vi "Review.vi"() -> ()   [LabVIEW 2023]
uses:
  <vilib>/measure/madcrms.llb/Basic Averaged DC-RMS for N Chan.vi
  <vilib>/measure/NI_MAPro.lvlib
panel:
  out "Mains Request":sgl
  out "Bus Current Load Demand":dbl
  out "Bus Voltage RMS/100":dbl
  out "Bus Current Demand to SM":dynamicdata(graph)
  out "Battery Charge Sw":bool
  out "Battery Discharge Sw":bool
  out "LoadSw3":bool
  out "LoadSw2":bool
  out "LoadSw1":bool
  out "SM PV Current":dbl
  out "SM Wind Current":dbl
  out "Bus Current (rms)":dynamicdata(graph)
  out "Bus Voltage (rms)":dynamicdata(graph)
  out "Load 3":bool
  out "Load 2":bool
  out "Load 1":bool
  out "Charge Batt":bool
  out "Discharge Batt":bool
  out "Analog Input (Main Capacity 0-10V)":dynamicdata(graph)
  in  "stop":bool
  out "Voltage Dip Supply < Demand":dynamicdata(graph)
  out "240 Vrms Supply >=Demand":dynamicdata(graph)
  out "Capacity - Demand (current)":dynamicdata(graph)
  in  "Battery Charging Current":dbl
  in  "Battery Disharging Current":dbl
  in  "Load 3 Demand (current)":dbl
  in  "Load 2 Demand (current)":dbl
  in  "Load 1 Demand (current)":dbl
  out "Battery Charging Current":dynamicdata(graph)
  out "Load 3 Current":dynamicdata(graph)
  out "Load 2 Current":dynamicdata(graph)
  out "Load 1 Current":dynamicdata(graph)
  out "Battery Discharging Current (A rms)":dynamicdata(graph)
  out "Main Available Current (A rms)":dynamicdata(graph)
  out "PV Available Current (A rms)":dynamicdata(graph)
  out "Wind Available Current (A rms)":dynamicdata(graph)
  in  "Main capacity (current)":dbl
  in  "Max PV capacity (current)":dbl
  in  "Max wind capacity (current)":dbl
  out "Bus Voltage 240Vrms/100":dynamicdata(graph)
  # "Smart Meter Emulator Algorithm inputs and output status"
  # "Final Review Software using software algorithm and profile inputs - produces output file for submission  - by Russel Torah - 2021"
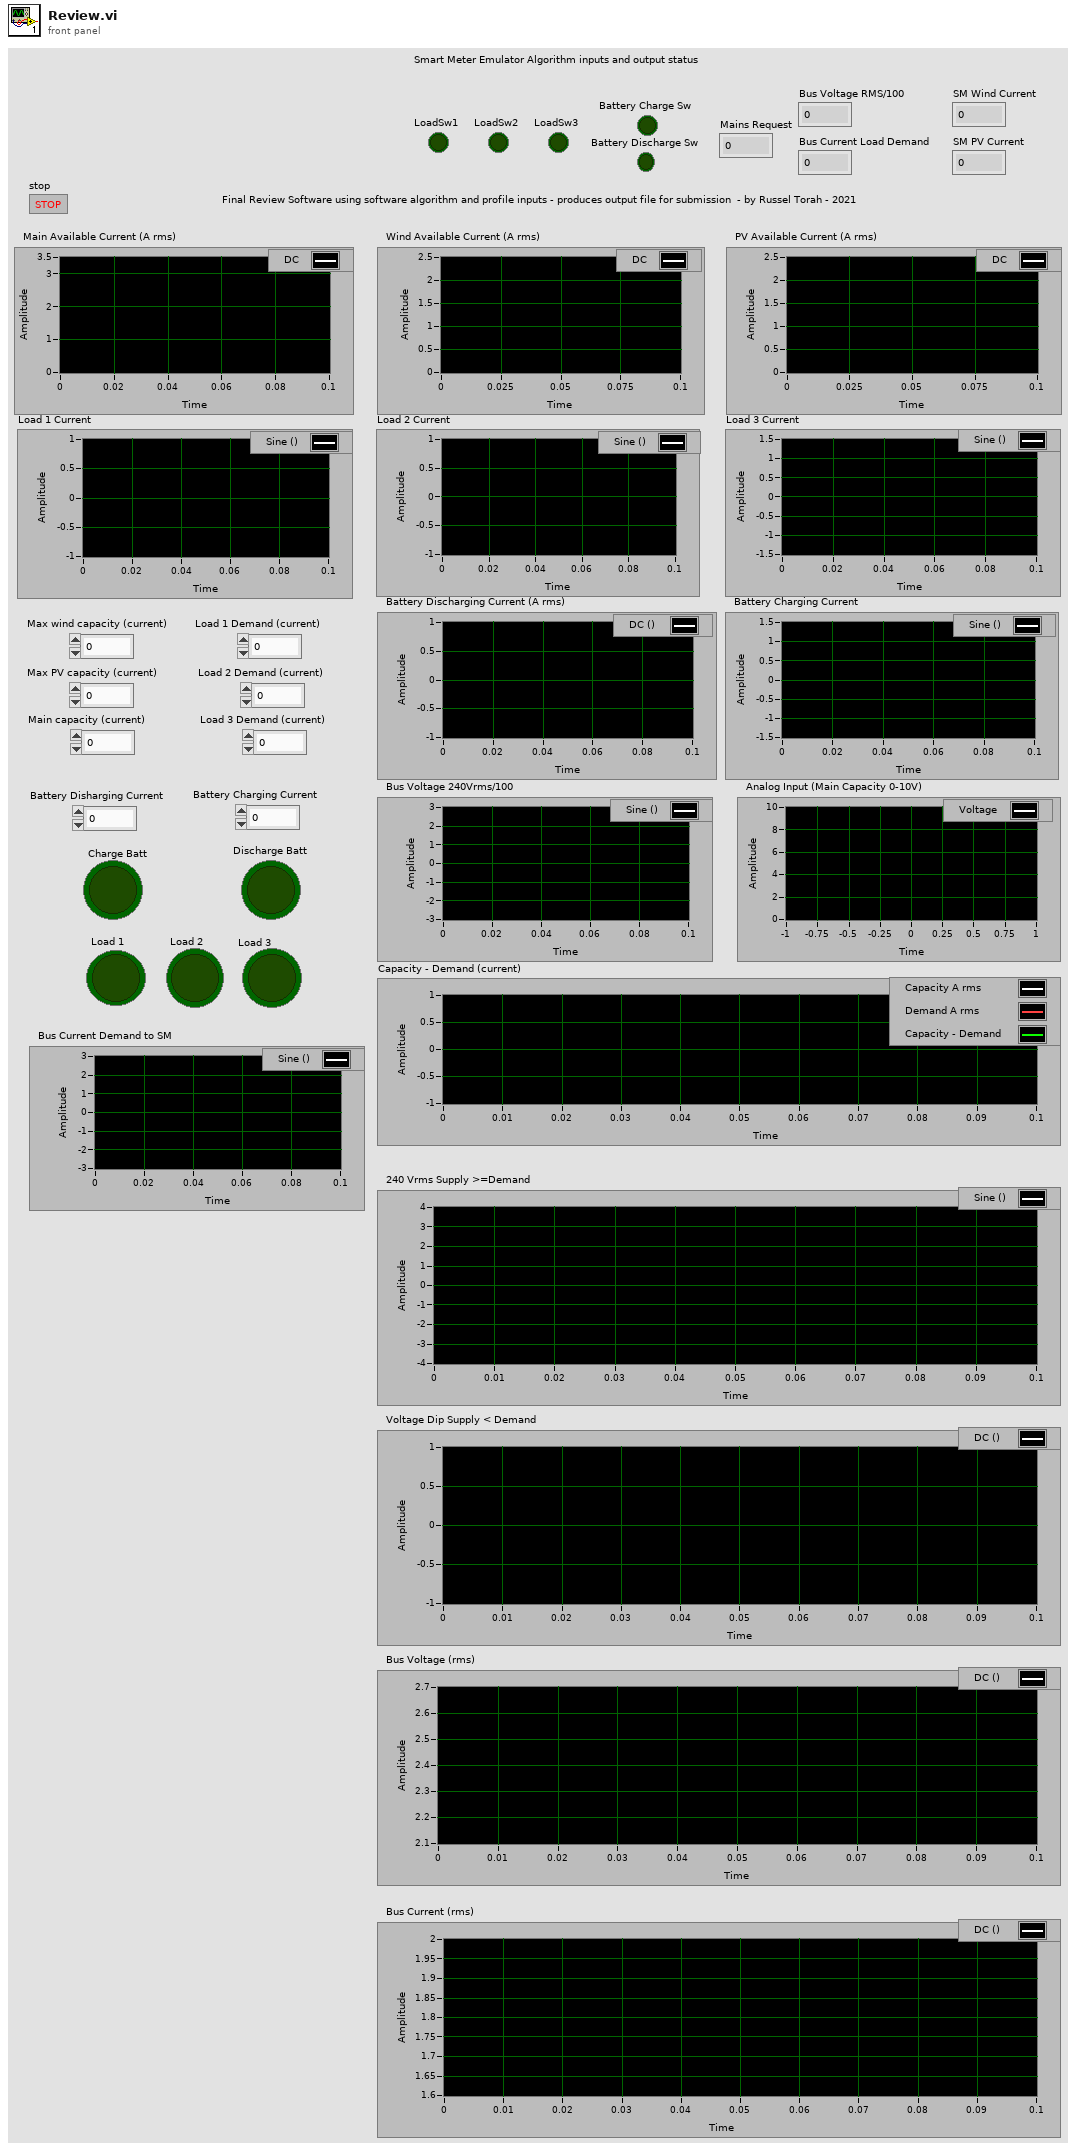
[diagram p1: front panel]
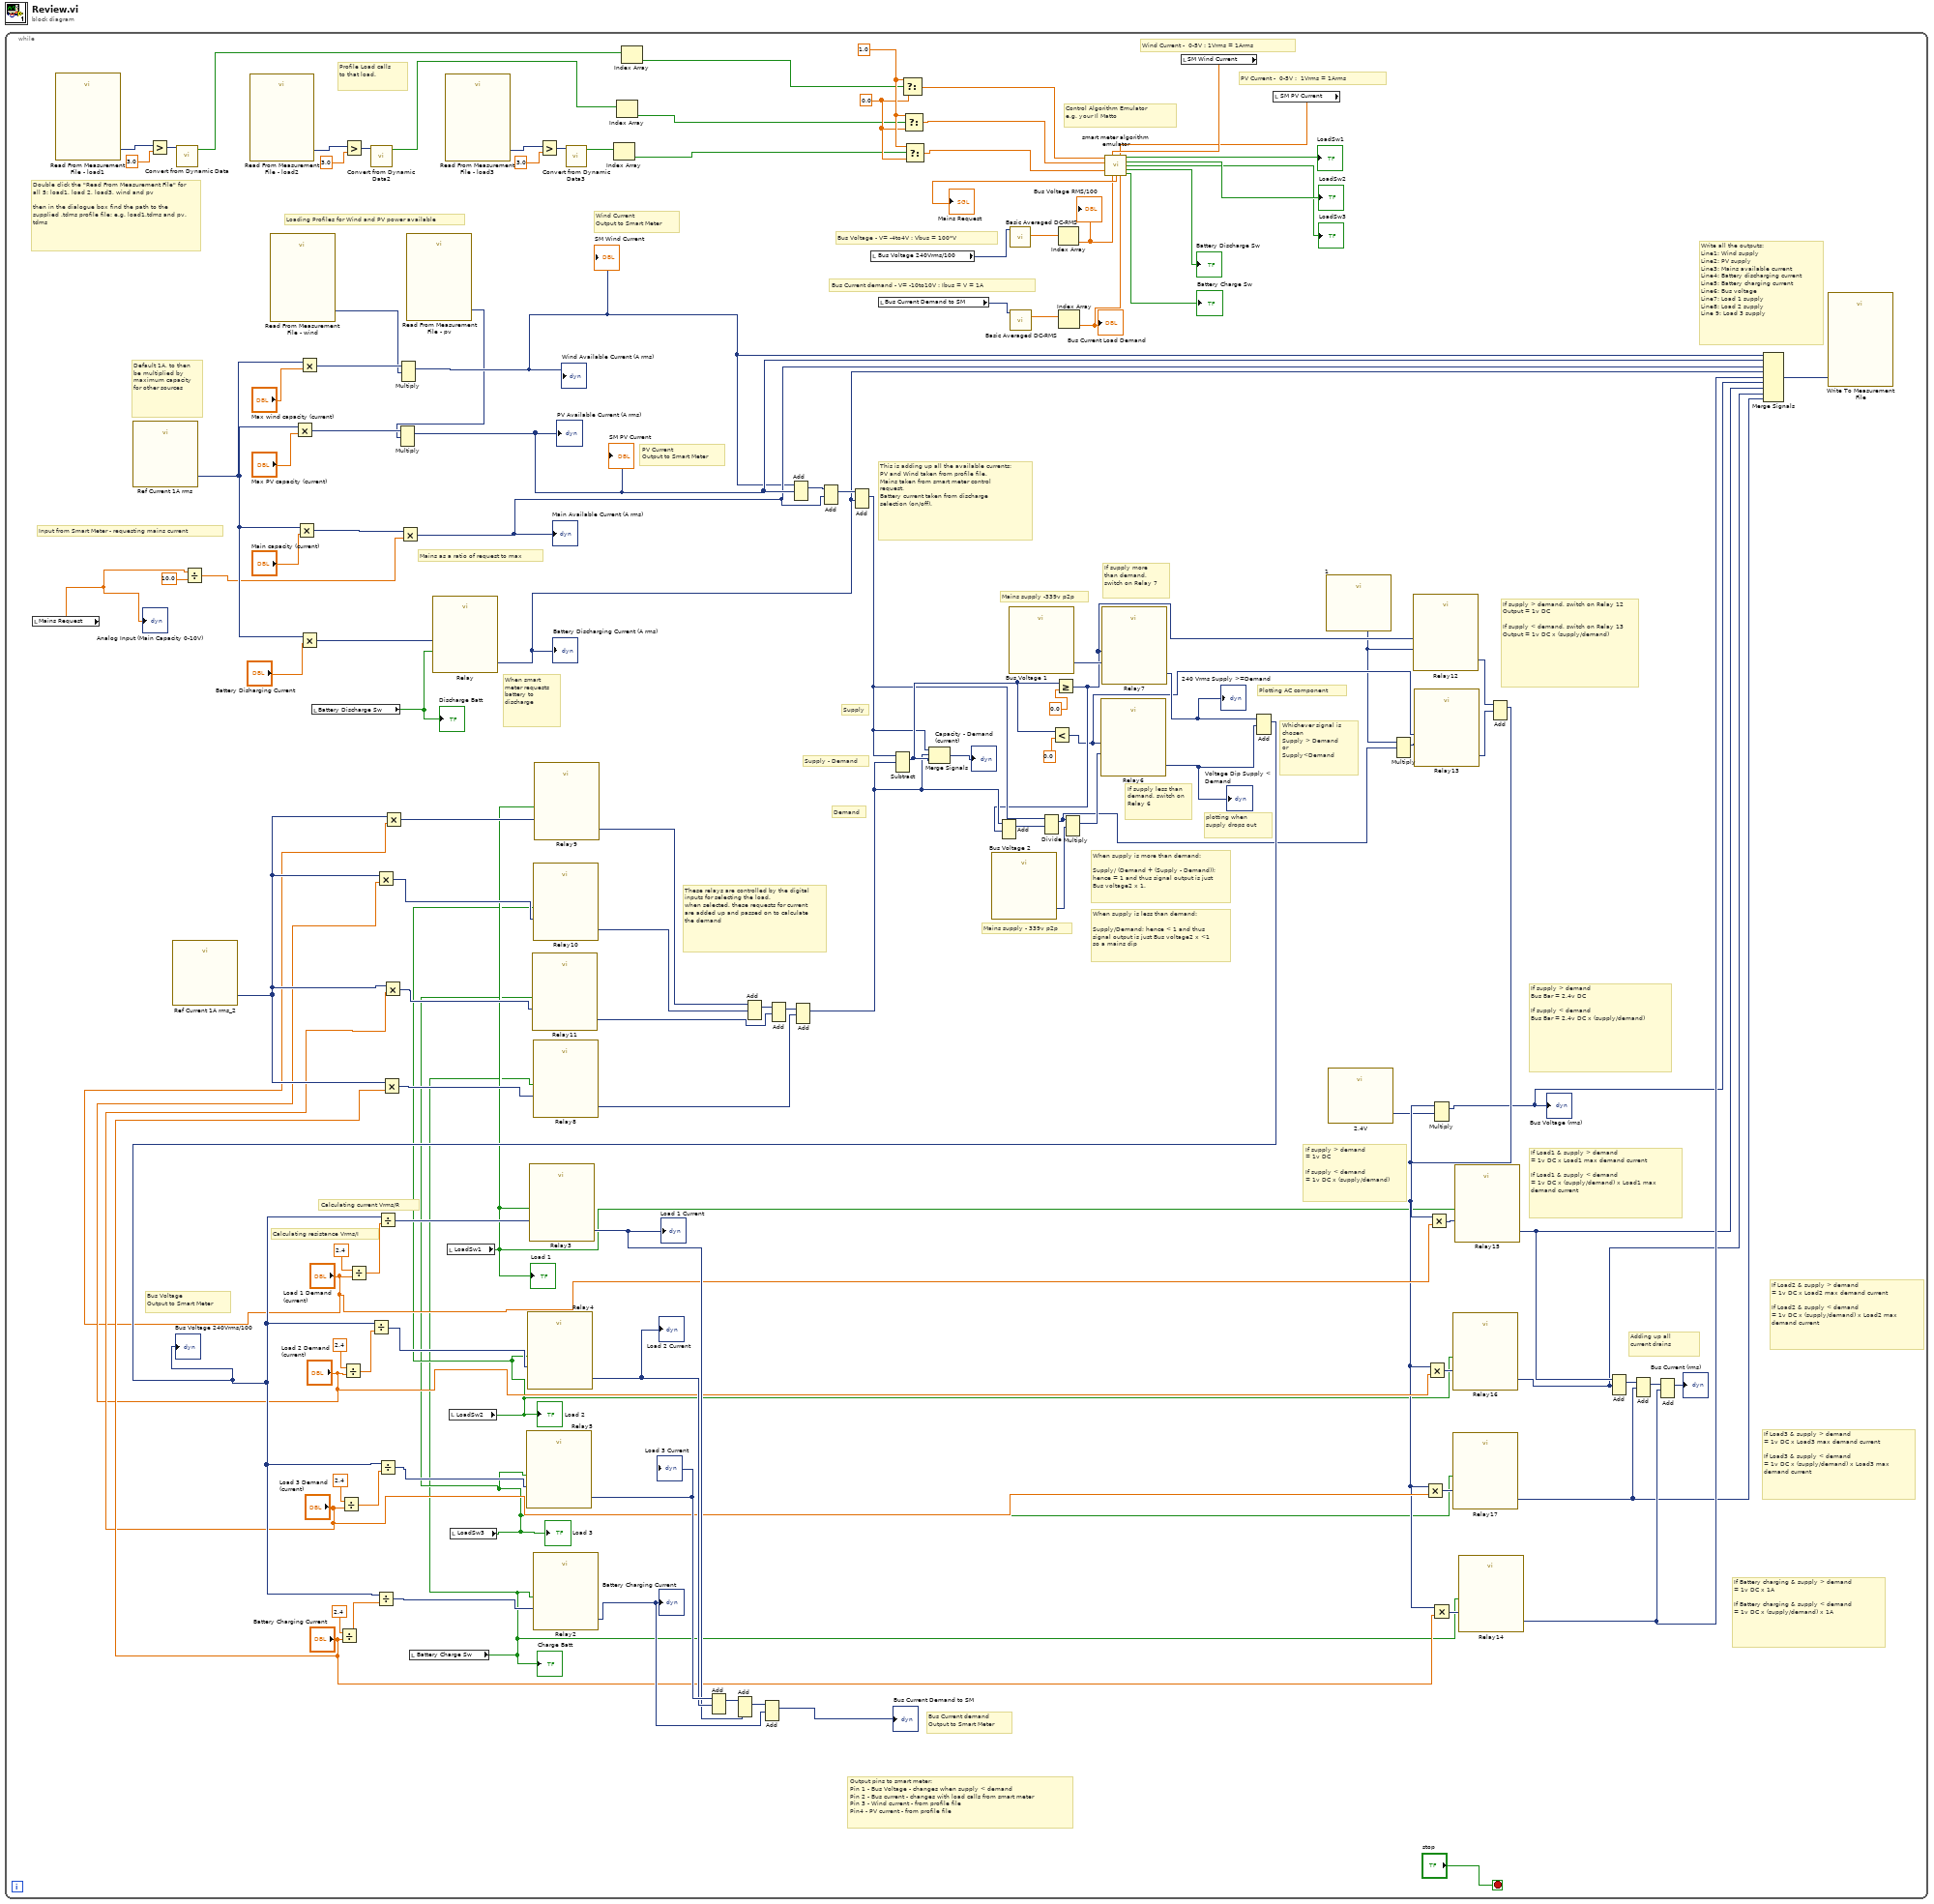
[diagram p0: block diagram]
diagram:
  n1 = while {
    stop <- "stop" stop-if-true
    w45 = 0.0 ("f")
    w46 = 1.0 ("t")
    # "Double click the \"Read From Measurement File\" for all 5: load1, load 2, load3, wind and pv\n\nthen in the dialogue box find the path to the supplied .tdms profile file: e.g. load1.tdms and pv.tdms"
    # "Bus Current demand - V= -10to10V : Ibus = V = 1A"
    # "Bus Voltage - V= -4to4V : Vbus = 100*V"
    # "Wind Current -  0-5V : 1Vrms = 1Arms"
    # "PV Current -  0-5V :  1Vrms = 1Arms"
    # "PV Current\nOutput to Smart Meter"
    # "Wind Current\nOutput to Smart Meter"
    # "Bus Current demand\nOutput to Smart Meter"
    # "Bus Voltage\nOutput to Smart Meter"
    # "Control Algorithm Emulator\ne.g. your Il Matto"
    # "Loading Profiles for Wind and PV power available"
    # "Profile Load calls\nto that load."
    # "Plotting AC component"
    # "plotting when supply drops out"
    # "Output pins to smart meter:\nPin 1 - Bus Voltage - changes when supply < demand\nPin 2 - Bus current - changes with load calls from smart meter\nPin 3 - Wind current - from profile file\nPin4 - PV current - from profile file"
    # "When smart meter requests battery to discharge"
    # "Mains as a ratio of request to max"
    # "Write all the outputs:\nLine1: Wind supply\nLine2: PV supply\nLine3: Mains available current\nLine4: Battery discharging current\nLine5: Battery charging current\nLine6: Bus voltage\nLine7: Load 1 supply\nLine8: Load 2 supply\nLine 9: Load 3 supply"
    # "Adding up all current drains"
    # "If Battery charging & supply > demand\n= 1v DC x 1A\n\nIf Battery charging & supply < demand\n= 1v DC x (supply/demand) x 1A"
    # "If Load3 & supply > demand\n= 1v DC x Load3 max demand current\n\nIf Load3 & supply < demand\n= 1v DC x (supply/demand) x Load3 max demand current"
    # "If Load2 & supply > demand\n= 1v DC x Load2 max demand current\n\nIf Load2 & supply < demand\n= 1v DC x (supply/demand) x Load2 max demand current"
    # "If Load1 & supply > demand\n= 1v DC x Load1 max demand current\n\nIf Load1 & supply < demand\n= 1v DC x (supply/demand) x Load1 max demand current"
    # "If supply > demand\n= 1v DC\n\nIf supply < demand\n= 1v DC x (supply/demand)"
    # "If supply > demand\nBus Bar = 2.4v DC\n\nIf supply < demand\nBus Bar = 2.4v DC x (supply/demand)"
    # "If supply > demand, switch on Relay 12\nOutput = 1v DC\n\nIf supply < demand, switch on Relay 13\nOutput = 1v DC x (supply/demand)"
    # "Whichever signal is chosen\nSupply > Demand\nor\nSupply<Demand"
    # "When supply is less than demand:\n\nSupply/Demand; hence < 1 and thus signal output is just Bus voltage2 x <1 so a mains dip"
    # "When supply is more than demand:\n\nSupply/ (Demand + (Supply - Demand)); hence = 1 and thus signal output is just Bus voltage2 x 1."
    # "Demand"
    # "Supply"
    # "If supply less than demand, switch on Relay 6"
    # "If supply more than demand, switch on Relay 7"
    # "Mains supply - 339v p2p"
    # "Mains supply -339v p2p"
    # "Supply - Demand"
    # "Calculating current Vrms/R"
    # "Calculating resistance Vrms/I"
    # "These relays are controlled by the digital inputs for selecting the load.\nwhen selected, these requests for current are added up and passed on to calculate the demand"
    # "Default 1A, to then be multiplied by maximum capacity for other sources"
    # "Input from Smart Meter - requesting mains current"
    # "This is adding up all the available currents:\nPV and Wind taken from profile file.\nMains taken from smart meter control request.\nBattery current taken from discharge selection (on/off)."
    n2 = local read "Mains Request"() -> (w31:sgl)
    "Analog Input (Main Capacity 0-10V)" <- w31
    n3 = call "Read From Measurement File - load1"() -> ("Signals"=w15:dynamicdata)  [unwired: 6 in, 5 out]
    n4 = call "Ref Current 1A rms"() -> ("DC"=w118:dynamicdata)  [unwired: 14 in, 1 out]
    n5 = Greater?(x=w15, y=3.0) -> (0:w16:dynamicdata)
    n6 = call "Ref Current 1A rms_2"() -> ("DC"=w78:dynamicdata)  [unwired: 14 in, 1 out]
    n7 = call "Convert from Dynamic Data"("Dynamic Data Type"=w16) -> ("Array"=w3:bool[])  [unwired: 3 in]
    n8 = Divide(x=w31, y=10.0) -> (x/y=w87:dbl)
    n9 = call "Read From Measurement File - load2"() -> ("Signals"=w12:dynamicdata)  [unwired: 6 in, 5 out]
    n10 = call "Read From Measurement File - wind"() -> ("Signals"=w19:dynamicdata)  [unwired: 6 in, 5 out]
    n11 = Multiply(x=w118, y="Max PV capacity (current)") -> (x*y=w127:dynamicdata)
    n12 = Multiply(x=w118, y="Main capacity (current)") -> (x*y=w126:dynamicdata)
    n13 = Multiply(x=w118, y="Max wind capacity (current)") -> (x*y=w128:dynamicdata)
    n14 = Multiply(x=w118, y="Battery Disharging Current") -> (x*y=w125:dynamicdata)
    n15 = local read "Battery Discharge Sw"() -> (w27:bool)
    "Discharge Batt" <- w27
    n16 = Divide(x=2.4, y="Battery Charging Current") -> (x/y=w106:dbl)
    n17 = Divide(x=2.4, y="Load 3 Demand (current)") -> (x/y=w108:dbl)
    n18 = Divide(x=2.4, y="Load 2 Demand (current)") -> (x/y=w111:dbl)
    n19 = Greater?(x=w12, y=3.0) -> (0:w13:dynamicdata)
    n20 = Divide(x=2.4, y="Load 1 Demand (current)") -> (x/y=w114:dbl)
    n21 = call "Convert from Dynamic Data2"("Dynamic Data Type"=w13) -> ("Array"=w5:bool[])  [unwired: 3 in]
    n22 = Multiply(x=w78, y="Load 2 Demand (current)") -> (x*y=w101:dynamicdata)
    n23 = Multiply(x=w78, y="Battery Charging Current") -> (x*y=w99:dynamicdata)
    n24 = Multiply(x=w78, y="Load 3 Demand (current)") -> (x*y=w100:dynamicdata)
    n25 = Multiply(x=w78, y="Load 1 Demand (current)") -> (x*y=w102:dynamicdata)
    n26 = Multiply(1:w19, 2:w128) -> (0:w41:dynamicdata)  [unwired: 1 in, 1 out]
    "Wind Available Current (A rms)" <- w41
    "SM Wind Current" <- w41
    n27 = Multiply(x=w126, y=w87) -> (x*y=w73:dynamicdata)
    "Main Available Current (A rms)" <- w73
    n28 = call "Read From Measurement File - pv"() -> ("Signals"=w18:dynamicdata)  [unwired: 6 in, 5 out]
    n29 = Multiply(1:w18, 2:w127) -> (0:w74:dynamicdata)  [unwired: 1 in, 1 out]
    "PV Available Current (A rms)" <- w74
    "SM PV Current" <- w74
    n30 = local read "Battery Charge Sw"() -> (w28:bool)
    "Charge Batt" <- w28
    n31 = call "Relay"("Enable"=w27, "Signals"=w125) -> ("Result"=w72:dynamicdata)  [unwired: 8 in, 1 out]
    "Battery Discharging Current (A rms)" <- w72
    n32 = call "Read From Measurement File - load3"() -> ("Signals"=w9:dynamicdata)  [unwired: 6 in, 5 out]
    n33 = local read "LoadSw1"() -> (w37:bool)
    "Load 1" <- w37
    n34 = local read "LoadSw2"() -> (w30:bool)
    "Load 2" <- w30
    n35 = local read "LoadSw3"() -> (w29:bool)
    "Load 3" <- w29
    n36 = call "Relay11"("Enable"=w29, "Signals"=w100) -> ("Result"=w96:dynamicdata)  [unwired: 8 in, 1 out]
    n37 = call "Relay10"("Enable"=w30, "Signals"=w101) -> ("Result"=w97:dynamicdata)  [unwired: 8 in, 1 out]
    n38 = call "Relay8"("Enable"=w28, "Signals"=w99) -> ("Result"=w95:dynamicdata)  [unwired: 8 in, 1 out]
    n39 = call "Relay9"("Enable"=w37, "Signals"=w102) -> ("Result"=w98:dynamicdata)  [unwired: 8 in, 1 out]
    n40 = Greater?(x=w9, y=3.0) -> (0:w10:dynamicdata)
    n41 = call "Convert from Dynamic Data3"("Dynamic Data Type"=w10) -> ("Array"=w6:bool[])  [unwired: 3 in]
    n42 = Index Array(array=w6) -> (element=w7:bool)  [unwired: 1 in]
    n43 = Index Array(array=w5) -> (element=w4:bool)  [unwired: 1 in]
    n44 = Index Array(array=w3) -> (element=w2:bool)  [unwired: 1 in]
    n45 = Add(1:w97, 2:w98) -> (0:w121:dynamicdata)  [unwired: 1 in, 1 out]
    n46 = Add(1:w96, 2:w121) -> (0:w120:dynamicdata)  [unwired: 1 in, 1 out]
    n47 = Add(1:w74, 2:w41) -> (0:w123:dynamicdata)  [unwired: 1 in, 1 out]
    n48 = Add(1:w95, 2:w120) -> (0:w75:dynamicdata)  [unwired: 1 in, 1 out]
    n49 = Add(1:w73, 2:w123) -> (0:w122:dynamicdata)  [unwired: 1 in, 1 out]
    n50 = Add(1:w72, 2:w122) -> (0:w76:dynamicdata)  [unwired: 1 in, 1 out]
    n51 = local read "Bus Voltage 240Vrms/100"() -> (w24:dynamicdata)
    n52 = local read "Bus Current Demand to SM"() -> (w22:dynamicdata)
    n53 = Subtract(1:w75, 2:w76) -> (0:w77:dynamicdata)  [unwired: 1 in, 1 out]
    n54 = Select(t=w46, s=w2, f=w45) -> (s? t:f=w44:dbl)
    n55 = Select(t=w46, s=w4, f=w45) -> (s? t:f=w43:dbl)
    n56 = Select(t=w46, s=w7, f=w45) -> (s? t:f=w42:dbl)
    n57 = Merge Signals(w76, w75, w77) -> (→"Capacity - Demand (current)":dynamicdata)
    n58 = call "Bus Voltage 2"() -> ("Sine"=w103:dynamicdata)  [unwired: 14 in, 1 out]
    n59 = call "Bus Voltage 1"() -> ("Sine"=w94:dynamicdata)  [unwired: 14 in, 1 out]
    n60 = call-poly <vilib>:"Basic Averaged DC-RMS.vi"("signals in"=w24) -> ("RMS values"=w25:dbl[])  [unwired: 7 in, 3 out]
    n61 = call-poly <vilib>:"Basic Averaged DC-RMS.vi"("signals in"=w22) -> ("RMS values"=w23:dbl[])  [unwired: 7 in, 3 out]
    n62 = Less?(x=w77, y=0.0) -> (x < y?=w70:dynamicdata)
    n63 = Greater Or Equal?(x=w77, y=0.0) -> (x >= y?=w71:dynamicdata)
    n64 = Add(1:w71, 2:w75) -> (0:w91:dynamicdata)  [unwired: 1 in, 1 out]
    n65 = Divide(1:w91, 2:w76) -> (0:w67:dynamicdata)  [unwired: 1 in, 1 out]
    n66 = Index Array(array=w25) -> (element=w21:dbl)  [unwired: 1 in]
    "Bus Voltage RMS/100" <- w21
    n67 = Index Array(array=w23) -> (element=w20:dbl)  [unwired: 1 in]
    "Bus Current Load Demand" <- w20
    n68 = Multiply(1:w103, 2:w67) -> (0:w93:dynamicdata)  [unwired: 1 in, 1 out]
    n69 = call "Relay6"("Enable"=w70, "Signals"=w93) -> ("Result"=w92:dynamicdata)  [unwired: 8 in, 1 out]
    "Voltage Dip Supply < Demand" <- w92
    n70 = call "Relay7"("Enable"=w71, "Signals"=w94) -> ("Result"=w90:dynamicdata)  [unwired: 8 in, 1 out]
    "240 Vrms Supply >=Demand" <- w90
    n71 = local read "SM Wind Current"() -> (w40:dbl)
    n72 = Add(1:w92, 2:w90) -> (0:w89:dynamicdata)  [unwired: 1 in, 1 out]
    "Bus Voltage 240Vrms/100" <- w89
    n73 = Divide(x=w89, y=w111) -> (x/y=w113:dynamicdata)
    n74 = Divide(x=w89, y=w106) -> (x/y=w107:dynamicdata)
    n75 = Divide(x=w89, y=w108) -> (x/y=w110:dynamicdata)
    n76 = Divide(x=w89, y=w114) -> (x/y=w116:dynamicdata)
    n77 = call "Relay5"("Enable"=w29, "Signals"=w110) -> ("Result"=w85:dynamicdata)  [unwired: 8 in, 1 out]
    "Load 3 Current" <- w85
    n78 = call "Relay4"("Enable"=w30, "Signals"=w113) -> ("Result"=w84:dynamicdata)  [unwired: 8 in, 1 out]
    "Load 2 Current" <- w84
    n79 = call "Relay3"("Enable"=w37, "Signals"=w116) -> ("Result"=w83:dynamicdata)  [unwired: 8 in, 1 out]
    "Load 1 Current" <- w83
    n80 = call "Relay2"("Enable"=w28, "Signals"=w107) -> ("Result"=w81:dynamicdata)  [unwired: 8 in, 1 out]
    "Battery Charging Current" <- w81
    n81 = Add(1:w84, 2:w85) -> (0:w86:dynamicdata)  [unwired: 1 in, 1 out]
    n82 = Add(1:w83, 2:w86) -> (0:w82:dynamicdata)  [unwired: 1 in, 1 out]
    n83 = Add(1:w81, 2:w82) -> (0:→"Bus Current Demand to SM":dynamicdata)  [unwired: 1 in, 1 out]
    n84 = local read "SM PV Current"() -> (w39:dbl)
    n85 = call "smart meter algorithm emulator.vi"("LoadCall1"=w44, "Wind available: 0 to 5 V DC"=w40, "PV available: 0 to 5 V DC"=w39, "LoadCall2"=w43, "LoadCall3"=w42, "Bus Voltage IN: -4 to 4 Vrms AC"=w21, "Bus Current IN: -10 to 10 Vrms AC"=w20) -> ("LoadSw1"=→"LoadSw1":bool, "LoadSw2"=→"LoadSw2":bool, "LoadSw3"=→"LoadSw3":bool, "Battery Discharge Sw"=→"Battery Discharge Sw":bool, "Mains Request"=→"Mains Request":sgl, "Battery Charge Sw"=→"Battery Charge Sw":bool)  [unwired: 3 in]
    n86 = call "1"() -> ("DC"=w68:dynamicdata)  [unwired: 14 in, 1 out]
    n87 = call "2.4V"() -> ("DC"=w55:dynamicdata)  [unwired: 14 in, 1 out]
    n88 = Multiply(1:w67, 2:w68) -> (0:w69:dynamicdata)  [unwired: 1 in, 1 out]
    n89 = call "Relay12"("Enable"=w71, "Signals"=w68) -> ("Result"=w66:dynamicdata)  [unwired: 8 in, 1 out]
    n90 = call "Relay13"("Enable"=w70, "Signals"=w69) -> ("Result"=w65:dynamicdata)  [unwired: 8 in, 1 out]
    n91 = Add(1:w65, 2:w66) -> (0:w56:dynamicdata)  [unwired: 1 in, 1 out]
    n92 = Multiply(x=w56, y="Load 3 Demand (current)") -> (x*y=w63:dynamicdata)
    n93 = Multiply(x=w56, y="Load 2 Demand (current)") -> (x*y=w62:dynamicdata)
    n94 = Multiply(x=w56, y="Load 1 Demand (current)") -> (x*y=w61:dynamicdata)
    n95 = Multiply(1:w55, 2:w56) -> (0:w50:dynamicdata)  [unwired: 1 in, 1 out]
    "Bus Voltage (rms)" <- w50
    n96 = Multiply(x=w56, y="Battery Charging Current") -> (x*y=w64:dynamicdata)
    n97 = call "Relay17"("Enable"=w29, "Signals"=w63) -> ("Result"=w47:dynamicdata)  [unwired: 8 in, 1 out]
    n98 = call "Relay16"("Enable"=w30, "Signals"=w62) -> ("Result"=w48:dynamicdata)  [unwired: 8 in, 1 out]
    n99 = call "Relay15"("Enable"=w37, "Signals"=w61) -> ("Result"=w49:dynamicdata)  [unwired: 8 in, 1 out]
    n100 = call "Relay14"("Enable"=w28, "Signals"=w64) -> ("Result"=w51:dynamicdata)  [unwired: 8 in, 1 out]
    n101 = Add(1:w48, 2:w49) -> (0:w54:dynamicdata)  [unwired: 1 in, 1 out]
    n102 = Add(1:w47, 2:w54) -> (0:w53:dynamicdata)  [unwired: 1 in, 1 out]
    n103 = Add(1:w51, 2:w53) -> (0:→"Bus Current (rms)":dynamicdata)  [unwired: 1 in, 1 out]
    n104 = Merge Signals(w41, w74, w73, w72, w51, w50, w49, w48, w47) -> (w8:dynamicdata)
    n105 = call "Write To Measurement File"("Signals"=w8) -> ()  [unwired: 16 in, 3 out]
  }
